vi "Read Data.vi"(8 "error in (no error)":errorcluster, 10 "COMMAND":string, 11 "VISA resource name in":refnum<visa-resource-name>) -> (0 "error out":errorcluster, 2 "Output":string, 3 "VISA resource name out":refnum<visa-resource-name>)   [LabVIEW 2010, in "DCP551.lvlib"]
uses:
  DCP551.lvlib
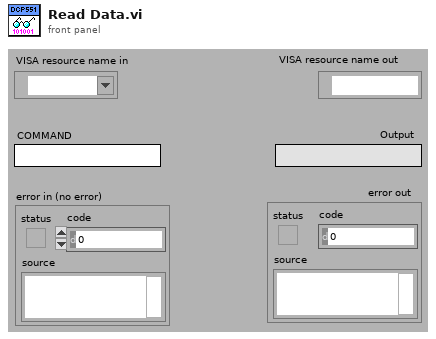
[diagram p1: front panel]
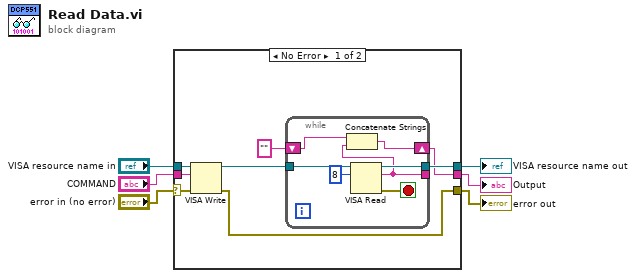
[diagram p0: block diagram]
diagram:
  n1 = case shown="No Error" "error in (no error)" {
    selector: "error in (no error)" -> [w9 w22]
    tunnel: "COMMAND" -> [w14 _]
    tunnel: "VISA resource name in" -> [w13 w23]
    tunnel: [w11 w23] -> w4
    tunnel: [w7 w22] -> w3
    tunnel: [w10 _] -> w2
    frame No Error {
      n2 = VISA Write(VISA resource name=w13, write buffer=w14, error in (no error)=w9) -> (VISA resource name out=w12:refnum<visa-resource-name>, error out=w7:errorcluster)  [unwired: 1 out]
      n3 = while {
        tunnel: [w21] -> w11
        tunnel: [w17] -> _
        tunnel: w12 -> [w19]
        shift-right: [w16] -> w10
        shift-left: "" -> [w15]
        stop <- w20 stop-if-true
        n4 = VISA Read(VISA resource name=w19, byte count=u32 8) -> (VISA resource name out=w21:refnum<visa-resource-name>, read buffer=w17:string, error out=w20:errorcluster)  [unwired: 1 in, 1 out]
        n5 = Concatenate Strings(w15, w17) -> (w16:string)
      }
    }
    frame Error {
    }
  }
  "error out" <- w3
  "VISA resource name out" <- w4
  "Output" <- w2
